vi "Open VI Panel.vi"(8 "error in":errorcluster, 11 "VI":refnum<vi>) -> (0 "error out":errorcluster)   [LabVIEW 2025, in "FlexiFlowInterface.lvlib"]
doc: "Open and activate the panel of the specified VI.\n_____\nCreated using DQMH Event Scripter 7.0.1.1316."
uses:
  FlexiFlowInterface/FlexiFlowInterface.lvlib
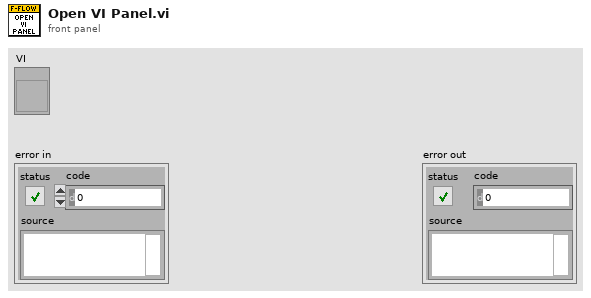
[diagram p1: front panel]
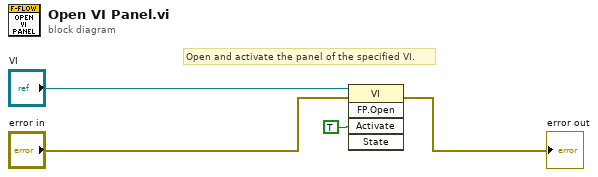
[diagram p0: block diagram]
diagram:
  # "Open and activate the panel of the specified VI."
  n1 = invoke class="VI" method="FP.Open"(reference="VI", error in="error in", "Activate"=TRUE ("Activate?")) -> (error out=→"error out":errorcluster)  [unwired: 2 in, 4 out]
